vi "number1-waveform generator.vi"() -> ()   [LabVIEW 2014]
panel:
  in  "Freq Scale":T1(ring)=enum."100"
  in  "Signal Type":enum16{"Triangular", "Squared", "Sine"}(ring)
  in  "Freq":dbl(knob)=5.606356388525899 scale=0.0..10.0
  in  "Amp":dbl(knob)=2.3806296682974613 scale=0.0..10.0
  out "Waveform Graph":ext[](graph)
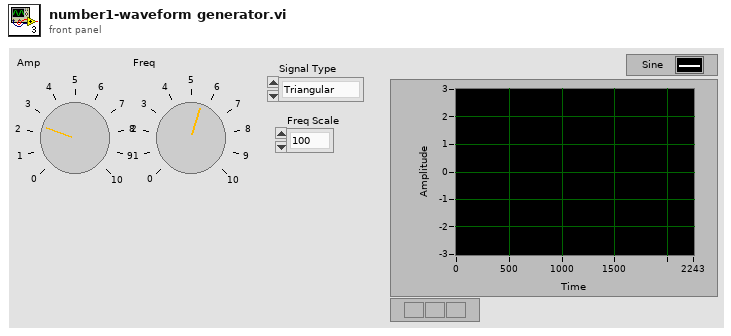
[diagram p1: front panel]
types:
  T1 = enum16{"10", "100", "1k", "10k", "100k", "1M", "10M"}
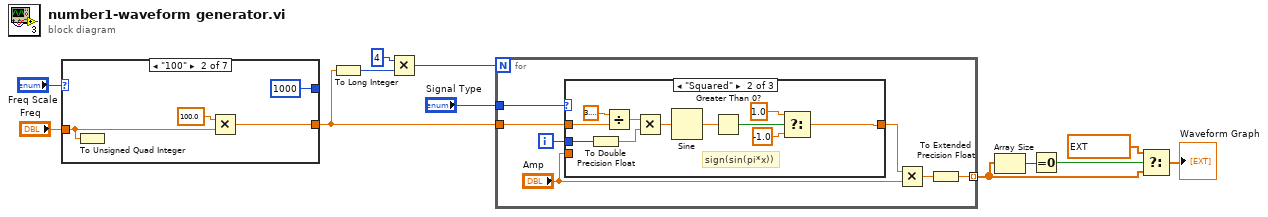
[diagram p0: block diagram]
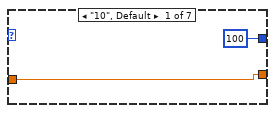
[diagram p2: hidden frame]
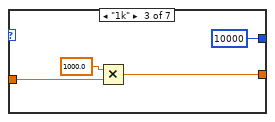
[diagram p3: hidden frame]
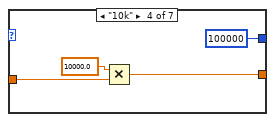
[diagram p4: hidden frame]
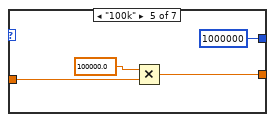
[diagram p5: hidden frame]
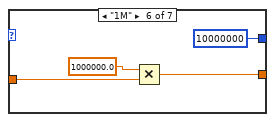
[diagram p6: hidden frame]
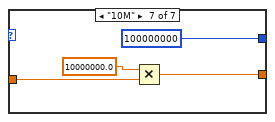
[diagram p7: hidden frame]
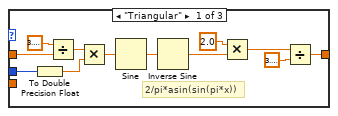
[diagram p8: hidden frame]
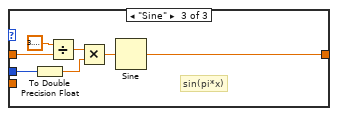
[diagram p9: hidden frame]
diagram:
  n1 = case shown="\"100\"" "Freq Scale" {
    tunnel: "Freq" -> [w14 w15 w21 w24 w29 w32 w36]
    tunnel: [w14 w18 w20 w25 w28 w33 w37] -> w9
    tunnel: [100 ("# of samples") 1000 ("# of samples") 10000 ("# of samples") 100000 ("# of samples") 1000000 ("# of samples") 10000000 ("# of samples") 100000000 ("# of samples")] -> _
    frame "10", Default {
    }
    frame "100" {
      n2 = To Unsigned Quad Integer(1:w15) -> ()  [unwired: 1 out]
      n3 = Multiply(x=100.0, y=w15) -> (x*y=w18:dbl)
    }
    frame "1k" {
      n4 = Multiply(x=1000.0, y=w21) -> (x*y=w20:dbl)
    }
    frame "10k" {
      n5 = Multiply(x=10000.0, y=w24) -> (x*y=w25:dbl)
    }
    frame "100k" {
      n6 = Multiply(x=100000.0, y=w29) -> (x*y=w28:dbl)
    }
    frame "1M" {
      n7 = Multiply(x=1000000.0, y=w32) -> (x*y=w33:dbl)
    }
    frame "10M" {
      n8 = Multiply(x=10000000.0, y=w36) -> (x*y=w37:dbl)
    }
  }
  n9 = To Long Integer(number=w9) -> (32bit integer=w8:i32)
  n10 = Multiply(x=4, y=w8) -> (x*y=w6:i32)
  n11 = for {
    N: w6 -> [_]
    tunnel: "Signal Type" -> [w44]
    tunnel: w9 -> [w42]
    tunnel: [w39] -> w3 mode=indexing
    i -> [w43]
    n12 = case shown="\"Squared\"" w44 {
      tunnel: [w46 w62 w75] -> w45
      tunnel: w43 -> [w52 w63 w73]
      tunnel: w42 -> [w53 w64 w70]
      tunnel: "Amp" -> [_ _ _]
      frame "Triangular" {
        # "2/pi*asin(sin(pi*x))"
        n13 = To Double Precision Float(number=w52) -> (double precision float=w56:dbl)
        n14 = Divide(x=3.141592653589793, y=w53) -> (x/y=w54:dbl)
        n15 = Multiply(x=w54, y=w56) -> (x*y=w57:dbl)
        n16 = Sine(x=w57) -> (sin(x)=w51:dbl)
        n17 = Inverse Sine(1:w51) -> (0:w50:dbl)
        n18 = Multiply(x=2.0, y=w50) -> (x*y=w47:dbl)
        n19 = Divide(x=w47, y=3.141592653589793) -> (x/y=w46:dbl)
      }
      frame "Squared" {
        # "sign(sin(pi*x))"
        n20 = To Double Precision Float(number=w63) -> (double precision float=w67:dbl)
        n21 = Divide(x=3.141592653589793, y=w64) -> (x/y=w65:dbl)
        n22 = Multiply(x=w65, y=w67) -> (x*y=w68:dbl)
        n23 = Sine(x=w68) -> (sin(x)=w61:dbl)
        n24 = Greater Than 0?(x=w61) -> (x > 0?=w60:bool)
        n25 = Select(t=1.0, s=w60, f=-1.0) -> (s? t:f=w62:dbl)
      }
      frame "Sine" {
        # "sin(pi*x)"
        n26 = To Double Precision Float(number=w73) -> (double precision float=w72:dbl)
        n27 = Divide(x=3.141592653589793, y=w70) -> (x/y=w69:dbl)
        n28 = Multiply(x=w69, y=w72) -> (x*y=w74:dbl)
        n29 = Sine(x=w74) -> (sin(x)=w75:dbl)
      }
    }
    n30 = Multiply(x=w45, y="Amp") -> (x*y=w40:dbl)
    n31 = To Extended Precision Float(1:w40) -> (0:w39:ext)
  }
  n32 = Array Size(array=w3) -> (size(s)=w4:i32)
  n33 = Equal To 0?(x=w4) -> (x = 0?=w5:bool)
  n34 = Select(t=ext[] [0.0, 0.0], s=w5, f=w3) -> (s? t:f=→"Waveform Graph":ext[])
